vi "shell integration settings.vi"(8 "error in":errorcluster, 10 "Extended?":bool=TRUE) -> (0 "error out":errorcluster, 3 "cluster out":T1)   [LabVIEW 2023, in "User Interface.lvlib"]
uses:
  User Interface.lvlib
  Controls/registry settings cluster.ctl
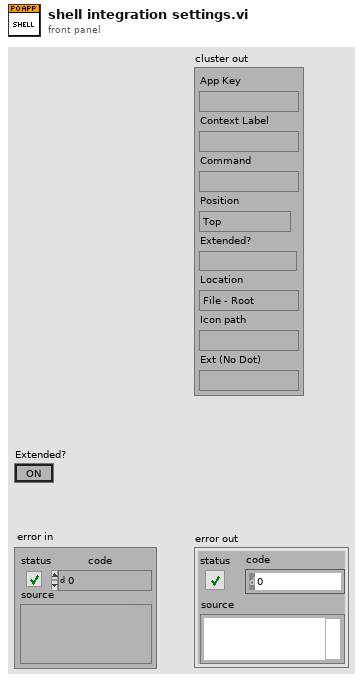
[diagram p1: front panel]
types:
  T1 = typedef "User Interface.lvlib/registry settings cluster.ctl" = cluster{"App Key":string, "Context Label":string, "Command":string, "Position":enum16{"Top", "Middle", "Bottom"}, "Extended?":bool, "Location":enum16{"File - Root", "Ext - Root", "Directory - Root", "File - Classes", "Ext - Classes", "Folder - Classes", "Dir Bak Gnd - Root"}, "Icon path":string, "Ext (No Dot)":string}
  T2 = enum16{"File - Root", "Ext - Root", "Directory - Root", "File - Classes", "Ext - Classes", "Folder - Classes"}
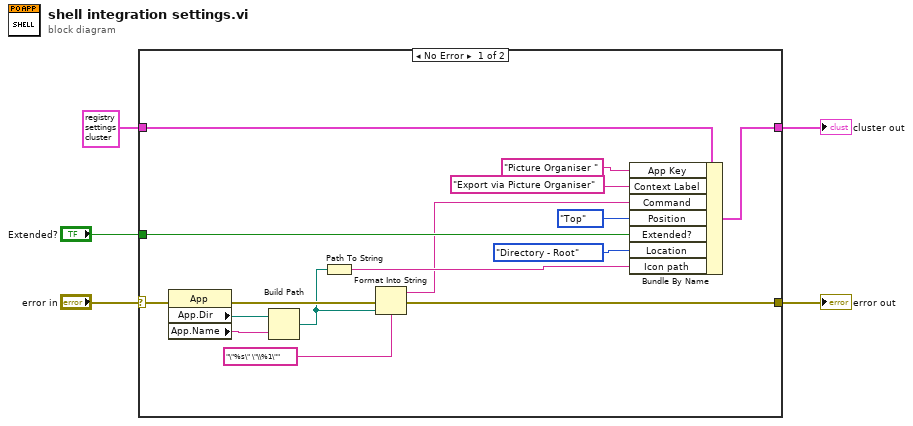
[diagram p0: block diagram]
diagram:
  n1 = case shown="No Error" "error in" {
    selector: "error in" -> [w6 w22]
    tunnel: [w20 w22] -> w5
    tunnel: "Extended?" -> [w16 _]
    tunnel: [w11 w23] -> w3
    tunnel: T1 {"App Key"="Test Key", "Context Label"="Test File Roottt", "Command"="Cmd", "Position"=enum."Middle", "Extended?"=FALSE, "Location"=enum."File - Root", "Icon path"="\"C:\\Users\\sajam\\LabVIEW Projects\\Personal projects\\Rename Extension\\Source Code\\rename.ico\"", "Ext (No Dot)"="Test"} ("Cluster") -> [w10 w23]
    frame No Error {
      n2 = property class="App"(error in=w6) -> (error out=w21:errorcluster, "App.Dir"=w7:path, "App.Name"=w8:string)  [unwired: 1 in, 1 out]
      n3 = Build Path(base path=w7, name or relative path=w8) -> (appended path=w18:path)
      n4 = Path To String(path=w18) -> (string=w19:string)
      n5 = Format Into String(format string="\"%s\" \"\\%1\"", error in=w21, w18) -> (resulting string=w14:string, error out=w20:errorcluster)  [unwired: 1 in]
      n6 = Bundle By Name(cluster=w10, "App Key"="Picture Organiser ", "Context Label"="Export via Picture Organiser", "Command"=w14, "Position"=enum16{"Top", "Middle", "Bottom"}."Top", "Extended?"=w16, "Location"=T2."Directory - Root", "Icon path"=w19) -> (w11:T1)
    }
    frame Error {
    }
  }
  "error out" <- w5
  "cluster out" <- w3
